vi "niDTS BT Tx Test Get Default Parameters.vi"(0 "Dummy Test Handle in":T9, 11 "error in (no error)":errorcluster) -> (4 "Dummy Test Handle out":T9, 8 "BT Tx Input Parameters":T1={"Channel"=0, "Data Rate "=1, "Dut Tx Power"=0.0, "External Attenuation (dB)"=[0.0, 0.0, 0.0, 0.0], "Auto Level"=FALSE, "Packet type"=enum."DH1", "Payload Pattern"=enum."PN9", "Burst Sync"=enum."PREamble", "BD ADDRESS"=0, "Packet Length, bytes"=37, "ModAcc Measurement Paramaters"={"ModAcc Enable"=FALSE, "CFO Enable"=FALSE, "Character Select"=enum."DF1", "Averages"=1, "Averaging Mode"=enum."RMS", "Measurement Length"=-1, "Measurement Offset"=0}, "OBW Measurement Parameters"={"OBW Enable"=FALSE, "OBW Averages"=1, "Averaging Type"=enum."RMS", "Measurement Interval Mode"=enum."AUTO", "Measurement Interval Length (sec)"=0.005}, "TXP Measurement Parameters"={"TXP Power Enable"=FALSE, "TXP Averages"=1, "Averaging Type"=enum."RMS"}, "IBE  Measurement Parameters"={"IBE Enable"=FALSE, "IBE Averages"=1, "Averaging Type"=enum."RMS", "Numbe of Channels"=11, "Channel Mode"=enum."Centered", "Measurement Interval Mode"=enum."AUTO", "Measurement Interval Length (sec)"=0.005}, "Trace Enable"=FALSE, "Trigger"={"MinQuietTimeDuration (sec)"=0.0001, "TriggerDelay (sec)"=0.0, "TriggerEdge"=enum."RISing", "TriggerSource"=enum."RF0", "TriggerThreshold (dB)"=-20.0, "TriggerTimeout (sec)"=10.0}} {"BD ADDRESS" max=16777215 format="%.0x"}, 15 "error out":errorcluster)   [LabVIEW 2014, in "niDTS BT.lvlib"]
uses:
  niDTS BT.lvlib
  Includes/niDTS BT Tx Test INC Handle.ctl
  Objects/BASE_class/niDTS BT Tx Test.lvclass
  Includes/niDTS BT Tx Test INC Parameters.ctl
  Includes/niDTS BT INC Packet Type.ctl
  Includes/niDTS BT Tx Test INC BD Payload Data.ctl
  Includes/niDTS BT Tx Test INC Modulation Characteristics.ctl
  Includes/niDTS BT INC OBW Measurement Parameters.ctl
  Includes/niDTS BT INC TXP Measurement Parameters.ctl
  EDR Tx Test/Includes/niDTS BT INC EDR IBE Measurement Parameters.ctl
  Includes/niDTS BT DUT INC Trigger.ctl
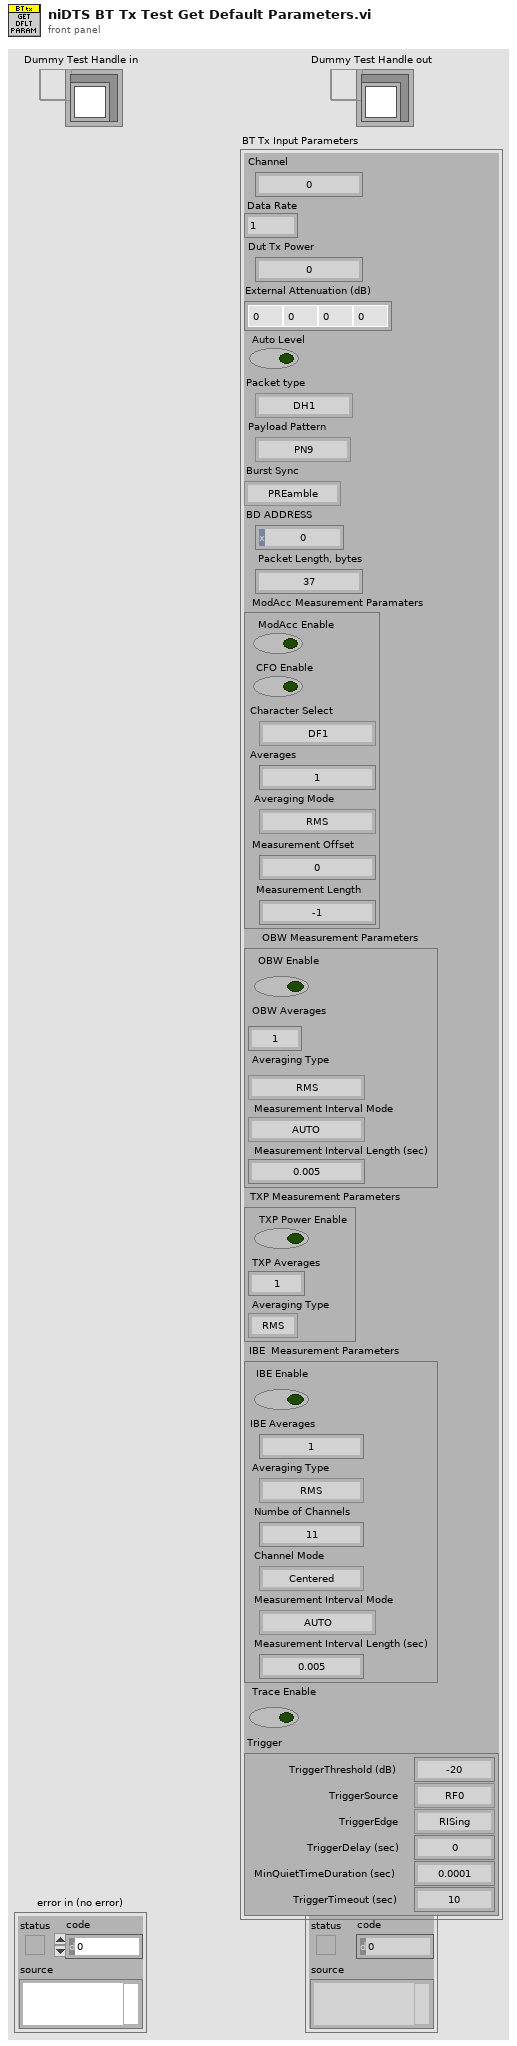
[diagram p1: front panel]
types:
  T1 = typedef "niDTS BT.lvlib/niDTS BT Tx Test INC Parameters.ctl" = cluster{"Channel":i32, "Data Rate ":i32, "Dut Tx Power":dbl, "External Attenuation (dB)":dbl[], "Auto Level":bool, "Packet type":T2, "Payload Pattern":T3, "Burst Sync":enum16{"NONE", "PREamble"}, "BD ADDRESS":u32, "Packet Length, bytes":i32, "ModAcc Measurement Paramaters":cluster{"ModAcc Enable":bool, "CFO Enable":bool, "Character Select":T4, "Averages":i32, "Averaging Mode":enum16{"RMS", "LOG", "SCALAR", "MAX", "MIN", "VECTOR"}, "Measurement Length":i32, "Measurement Offset":i32}, "OBW Measurement Parameters":T5, "TXP Measurement Parameters":T6, "IBE  Measurement Parameters":T7, "Trace Enable":bool, "Trigger":T8}
  T2 = typedef "niDTS BT.lvlib/niDTS BT INC Packet Type.ctl" = enum16{"NULL", "POLL", "FHS", "DM1", "DH1", "HV1", "HV2", "HV3", "EV3", "DV", "AUX1", "DM3", "DH3", "EV4", "EV5", "DM5", "DH5", "LE-TP"}
  T3 = typedef "niDTS BT.lvlib/niDTS BT Tx Test INC BD Payload Data.ctl" = enum16{"0", "1", "01", "00001111", "PN9", "AUTO"}
  T4 = typedef "niDTS BT.lvlib/niDTS BT Tx Test INC Modulation Characteristics.ctl" = enum16{"DF1", "DF2", "BOTH"}
  T5 = typedef "niDTS BT.lvlib/niDTS BT INC OBW Measurement Parameters.ctl" = cluster{"OBW Enable":bool, "OBW Averages":i32, "Averaging Type":enum16{"RMS", "LOG", "SCALAR", "MAX", "MIN", "VECTOR"}, "Measurement Interval Mode":enum16{"AUTO", "MANUAL"}, "Measurement Interval Length (sec)":dbl}
  T6 = typedef "niDTS BT.lvlib/niDTS BT INC TXP Measurement Parameters.ctl" = cluster{"TXP Power Enable":bool, "TXP Averages":i32, "Averaging Type":enum16{"RMS", "LOG", "SCALAR", "MAX", "MIN"}}
  T7 = typedef "niDTS BT.lvlib/niDTS BT INC EDR IBE Measurement Parameters.ctl" = cluster{"IBE Enable":bool, "IBE Averages":i32, "Averaging Type":enum16{"RMS", "LOG", "SCALAR", "MAX", "MIN", "VECTOR"}, "Numbe of Channels":i32, "Channel Mode":enum16{"InBand", "Centered"}, "Measurement Interval Mode":enum16{"AUTO", "MANUAL"}, "Measurement Interval Length (sec)":dbl}
  T8 = typedef "niDTS BT.lvlib/niDTS BT DUT INC Trigger.ctl" = cluster{"MinQuietTimeDuration (sec)":dbl, "TriggerDelay (sec)":dbl, "TriggerEdge":enum16{"RISing", "FALLing"}, "TriggerSource":enum16{"IMMediate", "RF0", "PFI0", "PFI1", "RTS0", "RTS1", "RTS2", "RTS3", "RTS4", "RTS5", "RTS6", "RTS7", "PXIStar", "SOFT"}, "TriggerThreshold (dB)":dbl, "TriggerTimeout (sec)":dbl}
  T9 = typedef "niDTS BT.lvlib/niDTS BT Tx Test INC Handle.ctl" = refnum<data-value>
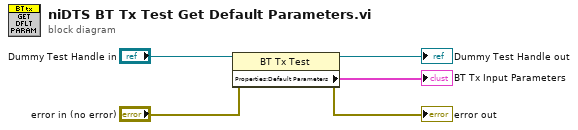
[diagram p0: block diagram]
diagram:
  n1 = property class="BT Tx Test"(reference="Dummy Test Handle in", error in="error in (no error)") -> (reference out=→"Dummy Test Handle out":T9, error out=→"error out":errorcluster, "Properties:Default Parameters"=→"BT Tx Input Parameters":T1)
